vi "optionsAcq_PDTemperatureMode.vi"(0 "reference":refnum<class "OSA.lvclass">, 2 "PD sensitivity mode":T1, 5 "error in (no error)":errorcluster, 9 "read/write":enum16{"read", "write"}(ring)) -> (14 "duplicate reference":refnum<class "OSA.lvclass">, 16 "PD sensitivity mode out":T1, 18 "PD senseMode implemented":bool, 19 "error out":errorcluster)   [LabVIEW 2010, in "OSA.lvclass"]
doc: "The OSA optical detectors in some models are cooled to improve the noise floor, (typically cooled at -30 degrees C for a reduction of thermal noise). However the cooling also restricts the upper wavelength range which is why a warm detector temperature mode can be selected to extend the range.\n[OSA200]"
uses:
  OSA.lvclass
  _misc/Thorlabs_FTS_misc.llb/PDTemperatureMode.ctl
  _dll/LVLib/FTSLib.lvlib
  OSA20X_misc.lvlib
panel:
  out "status":string
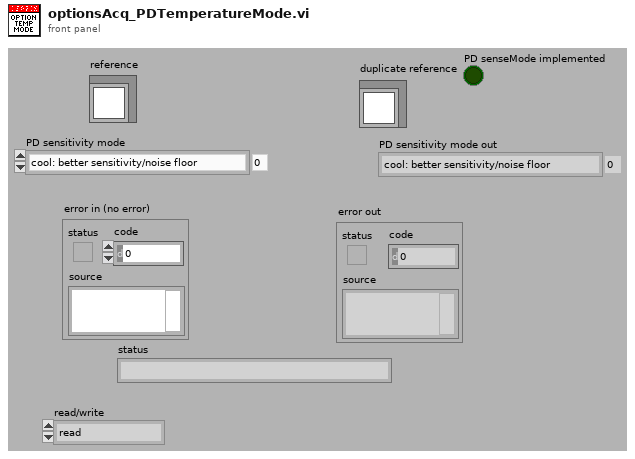
[diagram p1: front panel]
types:
  T1 = typedef "OSA20X_misc.lvlib/PDTemperatureMode.ctl" = enum16{"cool: better sensitivity/noise floor", "warm: extended wl range"}
  T2 = typedef "OSA.lvclass/ObjectAttributes.ctl" = cluster{"Stop":bool, "dataType":T3, "spectrometerIdx":u16, "buffer size interferogram":i32, "interferogram":cluster{"new":bool, "plot_x_ min":sgl, "plot_x_max":sgl, "plot_y_min":sgl, "plot_y_max":sgl, "Graph Intrfrgrm":T4, "timeStamp":u32, "signal (%)":dbl, "traces":cluster{"idx":u32, "broadBand":bool, "monoChromatic":bool, "peakToPeakSignal":dbl, "peakToPeakPos":dbl}[], "traces idx last":i32}, "spectrum":cluster{"new":bool, "plot_x_min":sgl, "plot_x_max":sgl, "plot_unit_x":T5, "plot_unit_y":T6, "plot_y_min":sgl, "plot_y_max":sgl, "Graph Spectrum":T4, "timeStamp":u32, "X_VAL_OPTIONS":enum16{"MIN_MAX", "ARRAY"}, "traces":cluster{"idx":u32}[], "traces idx last":i32}, "Thorlabs_OSA_64.lvclass:queue_action.ctlqueue ref":refnum<queue>, "action":T7, "plot zoom step":dbl, "buffer semaphore":T8, "acq stopped":bool, "dataType active":T3, "temperature (degr C)":sgl, "pressure (hPa)":sgl, "rel humidity (%)":sgl, "settings":cluster{"resolution":u16, "sensitivity":u16, "Average":bool, "average nr":u32, "apodisation":T9, "acq delay (ms)":u32, "airMesure":T10, "wmtr on":bool, "intfgrm_smooth_width":u16, "intfgrm_smooth_nrOfPasses":u16, "intfgrm_smooth":T11, "phaseCorrection":T12, "zeroFill":u8, "spectr_smooth":T11, "spectr_smooth_width":u16, "spectr_smooth_nrOfPasses":u16, "resolution (/cm)":sgl, "REF wavelength, (nm)":dbl, "gain_idx":u16, "gainAuto":bool, "gain_relative":dbl, "PD sensitivity mode":T1, "PD senseMode implemented":bool, "SensorTemperature implemented":bool, "SensorPressure implemented":bool, "SensorHumidity implemented":bool}, "peaks position":sgl[], "peaks width":sgl[], "peaks height":sgl[], "peaks max nr":u32, "peaks latest nr":i32, "peaks new":bool, "power":dbl, "power new":bool, "path":string, "wavelength (WNr)":dbl, "wavelength new":bool, "buffer size spectrum":i32, "status":string, "VI reference":refnum<vi>, "funcPointer":u64, "libraryPointer":u64, "singleAcquisition":bool, "coherenceLength (cm)":dbl, "coherenceLength new":bool, "spectrometer model":string, "spectrometer serial nr":string, "peaks thld left":sgl[], "peaks thld right":sgl[], "coherenceLength error (cm)":dbl, "ADC bits":u16, "peaks position centroid":sgl[], "peaks height centroid":sgl[], "OSA series":T13, "channel index spectrum":u16, "spectrometer rangeLow, (/cm)":dbl, "spectrometer rangeHigh, (/cm)":dbl, "channel index interferogram":u16}
  T3 = typedef "OSA.lvclass/acq_dataType.ctl" = enum16{"none", "interferogram", "spectrum"}
  T4 = typedef "OSA.lvclass/graph_intensity.ctl" = refnum<vi>
  T5 = typedef "OSA.lvclass/spectrum_x_unit.ctl" = enum16{"wavenr/cm", "THz", "eV", "nm_air", "nm_vac"}
  T6 = typedef "OSA.lvclass/y_unit.ctl" = enum16{"ADC counts", "dBm pwr absolute", "dBm pwr density", "mW pwr absolute", "mW pwr density"}
  T7 = typedef "OSA.lvclass/queue_action.ctl" = enum16{"none", "stop", "GUI_plotInterferogram", "GUI_plotSpectrum", "GUI_plotInterferogramRescale", "GUI_plotSpectrumRescale", "GUI_plotInterferogramReset", "GUI_plotSpectrumReset", "GUI_plotInterferogramAutoScaleY", "GUI_plotSpectrumAutoScaleY", "GUI_plotInterferogramZoomOut", "GUI_plotSpectrumZoomOut", "GUI_plotInterferogramPane", "GUI_plotSpectrumPane", "GUI_plotInterferogramZoomMouse", "GUI_plotSpectrumZoomMouse", "ENVIRONMENT temperature", "ENVIRONMENT pressure", "MODE_resolution set", "MODE_resolution get", "MODE_sensitivity set", "MODE_sensitivity get", "MODE_PDTemperature set", "MODE_PDTemperature get", "REBOOT/RESET firmware", "ACQASYNC_acquireSingleSpectrum", "ACQASYNC_continuous start", "ACQASYNC_continuous stop\n", "ACQASYNC_get last interferogram", "ACQASYNC_get last spectrum", "ACQASYNC_get last waveNr", "ACQOPT_interferogram smoothing set", "ACQOPT_interferogram smoothing get", "ACQOPT_spectrum smoothing set", "ACQOPT_spectrum smoothing get", "ACQOPT_apodisation type set", "ACQOPT_apodisation type get", "ACQOPT_phase correction type set", "ACQOPT_phase correction type get", "ACQOPT_acqIntervall_set", "ACQOPT_acqIntervall_get", "ACQOPT_average spectrum set", "ACQOPT_average spectrum get", "ACQOPT_rolling average set", "ACQOPT_rolling average get", "ACQOPT_zero fill factor set", "ACQOPT_zero fill factor get", "ACQOPT_cycle counting set", "ACQOPT_cycle counting get", "ACQOPT_air measure option set", "ACQOPT_air measure option get", "ACQOPT_gainLevel auto get", "ACQOPT_gainLevel auto set", "ACQOPT_gainLevel get", "ACQOPT_gainLevel set", "ACQOPT_getAll", "INSTRUMENT_PROPERTY_range_WaveNr_min", "INSTRUMENT_PROPERTY_range_WaveNr_max", "INSTRUMENT_PROPERTY_reference_wavelength_cm^-1", "INSTRUMENT_PROPERTY_samplesPerRefPeriod", "INSTRUMENT_PROPERTY_resolution_waveNrPercm", "INSTRUMENT_PROPERTY_availableGainLevels", "INSTRUMENT_PROPERTY_status", "CONVERT", "ANALYSE_POWER", "ANALYSE_PEAKS", "ANALYSE_WAVELENGTH", "ANALYSE_SPECTRUM", "ANALYSE_INTERFEROGRAM", "ANALYSE_COHERENCE_LENGTH", "MATH", "MATH_power", "MATH_peaks", "FILE", "miscellaneous"}
  T8 = typedef "Semaphore RefNum" = refnum<k1>
  T9 = typedef "OSA.lvclass/apodisation.ctl" = enum16{"NONE", "NORTON_BEER_WEAK", "NORTON_BEER_MEDIUM", "NORTON_BEER_STRONG", "TRIANGULAR", "COSINE", "HANN", "HAMMING", "BLACKMANHARRIS3", "BLACKMANHARRIS4", "GAUSSIAN"}
  T10 = typedef "OSA.lvclass/airMeasure.ctl" = enum16{"TEMPERATURE", "PRESSURE"}
  T11 = typedef "OSA20X_misc.lvlib/interferogram_smoothing.ctl" = enum16{"NONE", "BINOMIAL", "SAVITSKY_GOLAY", "FOURIER", "MOVING_AVERAGE", "GAUSSIAN"}
  T12 = typedef "OSA.lvclass/phaseCorrection.ctl" = enum16{"NONE", "MERTZ", "FORMAN", "MERTZ_FILE", "FORMAN_FILE", "FUTURE COMP."}
  T13 = typedef "OSA.lvclass/OSA_series.ctl" = enum16{"OSA200", "OSA300", "UNKNOWN"}
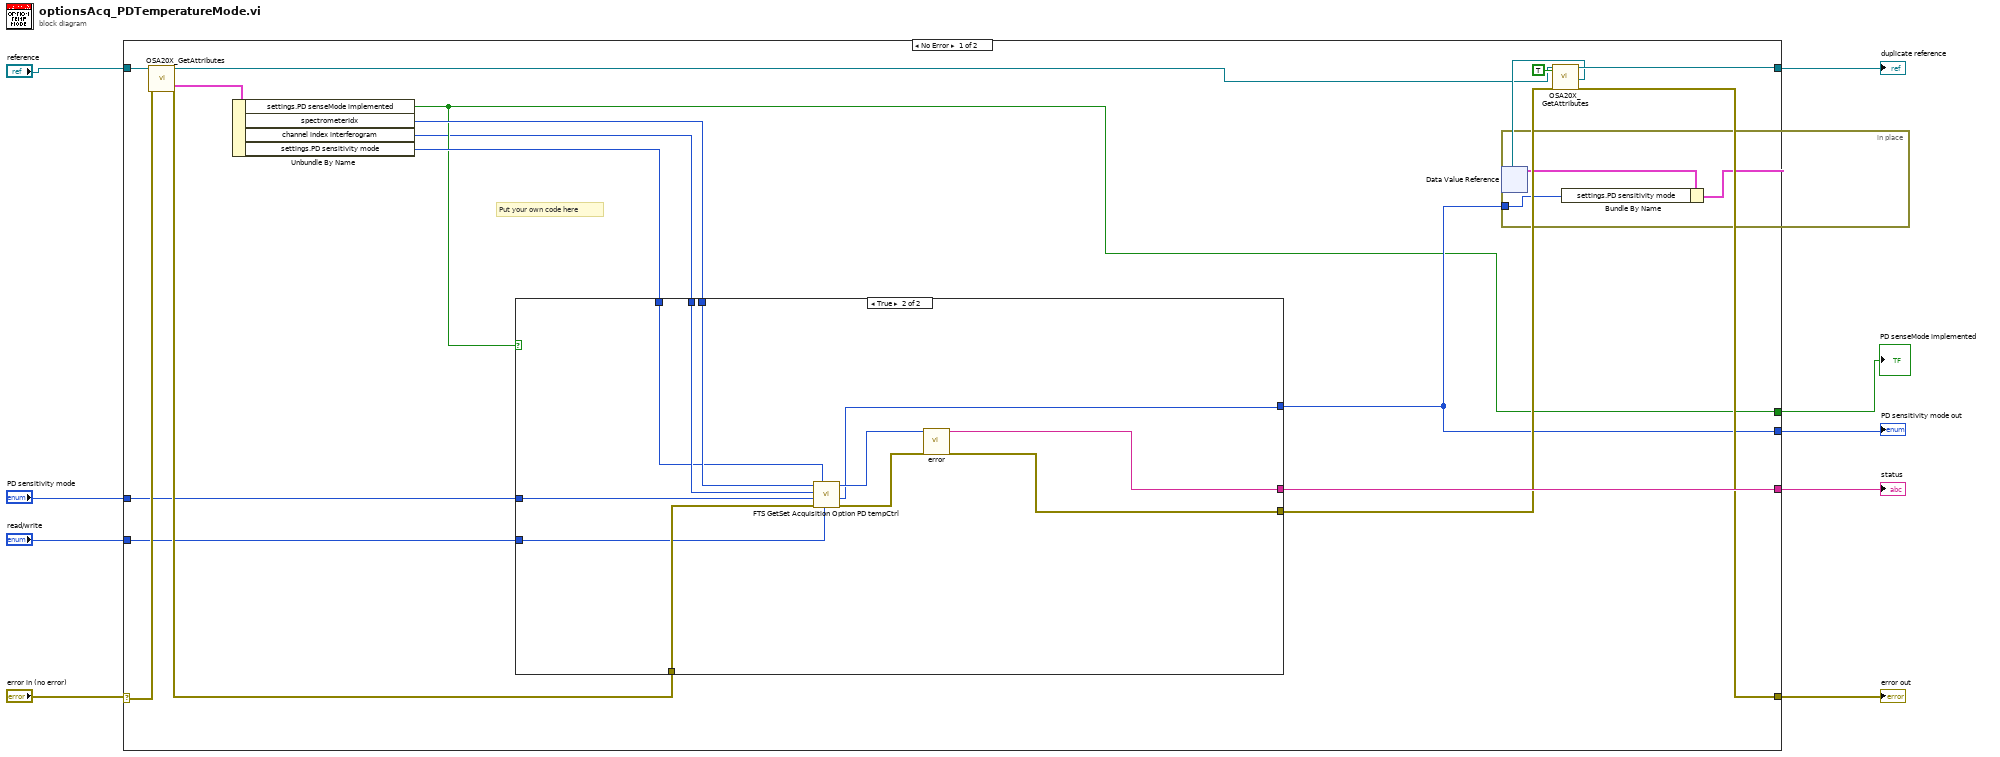
[diagram p0: block diagram]
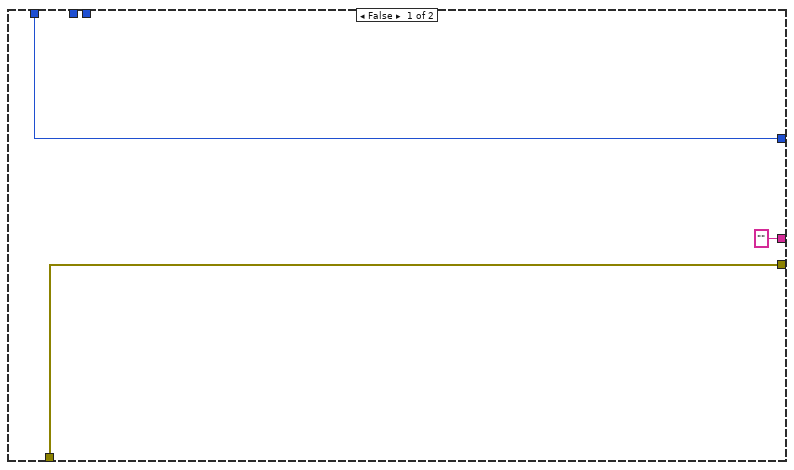
[diagram p2: hidden frame]
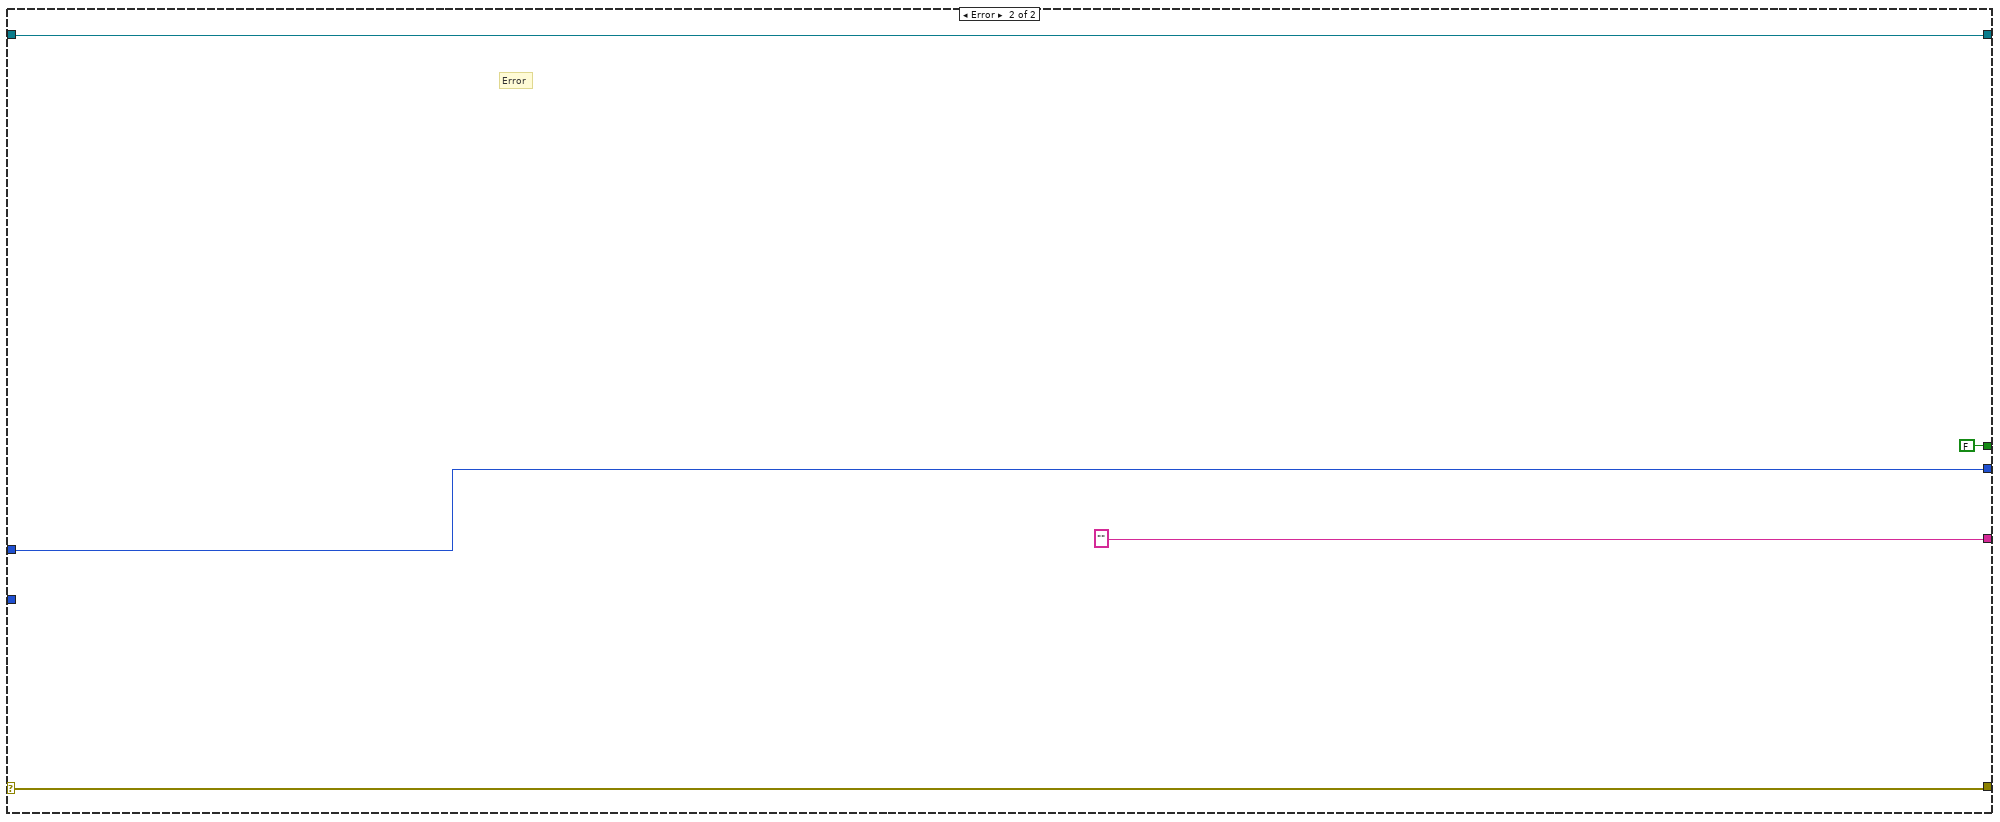
[diagram p3: hidden frame]
diagram:
  n1 = case shown="No Error" "error in (no error)" {
    selector: "error in (no error)" -> [w26 w48]
    tunnel: [w18 w48] -> w9
    tunnel: "reference" -> [w27 w49]
    tunnel: [w20 w49] -> w6
    tunnel: "PD sensitivity mode" -> [w21 w46]
    tunnel: [w24 "" ("status")] -> w4
    tunnel: "read/write" -> [w22 _]
    tunnel: [w13 w46] -> w2
    tunnel: [w11 FALSE ("PDTempCtrl_available")] -> w1
    frame No Error {
      # "Put your own code here"
      n2 = call "OSA20X_GetAttributes.vi"("reference in"=w27, "error in (no error)"=w26) -> ("reference out"=w12:refnum<class "OSA.lvclass">, "Data"=w15:T2, "error out"=w25:errorcluster)  [unwired: 14 in, 1 out]
      n3 = Unbundle By Name(w15) -> ("settings.PD senseMode implemented"=w11:bool, "spectrometerIdx"=w23:u16, "channel index interferogram"=w10:u16, "settings.PD sensitivity mode"=w17:T1)
      n4 = case shown="True" w11 {
        tunnel: w25 -> [w30 w39]
        tunnel: ["" ("status") w36] -> w24
        tunnel: w23 -> [_ w41]
        tunnel: w22 -> [_ w34]
        tunnel: w21 -> [_ w33]
        tunnel: [w30 w35] -> w19
        tunnel: w17 -> [w28 w32]
        tunnel: [w28 w31] -> w13
        tunnel: w10 -> [_ w40]
        frame False {
        }
        frame True {
          n5 = call "FTS GetSet Acquisition Option PD tempCtrl.vi"("read/write"=w34, "PD sensitivity mode Pre"=w32, "error in"=w39, "PD sensitivity mode write"=w33, "channel index interferogram"=w40, "spectrometerIdx"=w41) -> ("error out"=w37:errorcluster, "PD sensitivity mode out"=w31:T1, "status FTSLib"=w38:i32)  [unwired: 3 in]
          n6 = call "error.vi"("result code"=w38, "error in (no error)"=w37) -> ("status"=w36:string, "error out"=w35:errorcluster)  [unwired: 15 in, 1 out]
        }
      }
      n7 = call "OSA20X_GetAttributes.vi"("reference in"=w12, "OnlyGetDvrReference(False)"=TRUE, "error in (no error)"=w19) -> ("reference out"=w20:refnum<class "OSA.lvclass">, "DataRef"=w14:refnum<data-value>, "error out"=w18:errorcluster)  [unwired: 13 in, 1 out]
      n8 = in-place {
        in-place-border: w13 -> [w43]
        n9 = in-place-dvr #1(w14) -> (w44:T2)  [unwired: 1 out]
        n10 = Bundle By Name(cluster=w44, "settings.PD sensitivity mode"=w43) -> (w42:T2)
        n11 = in-place-dvr #1(w42) -> ()  [unwired: 2 out]
      }
    }
    frame Error {
      # "Error"
    }
  }
  "error out" <- w9
  "duplicate reference" <- w6
  "status" <- w4
  "PD sensitivity mode out" <- w2
  "PD senseMode implemented" <- w1
